vi "relay_block6.vi"(8 "error in":errorcluster, 11 "Modbus master in":refnum<class "Modbus Master.lvclass">) -> (0 "error out":errorcluster, 3 "Modbus master out":refnum<class "Modbus Master.lvclass">)   [LabVIEW 2020]
uses:
  <vilib>/NI/Modbus Library/API/Master/Modbus Master.lvclass
  C:/Program Files/National Instruments/LabVIEW 2020/vi.lib/NI/Modbus Library/API/Modbus API.lvclass
  <vilib>/NI/Modbus Library/API/Modbus API.lvclass/Modbus API.ctl
  <vilib>/NI/Modbus Library/Transmission Data Unit/Transmission Data Unit.lvclass/Transmission Data Unit.ctl
  <vilib>/NI/Modbus Library/Transmission Data Unit/Write Unit ID.vi
  <vilib>/NI/Modbus Library/API/Read Transmission Data Unit.vi
  <vilib>/NI/Modbus Library/API/Write Transmission Data Unit.vi
  status/emergency stop.vi
panel:
  out "current time":timestamp
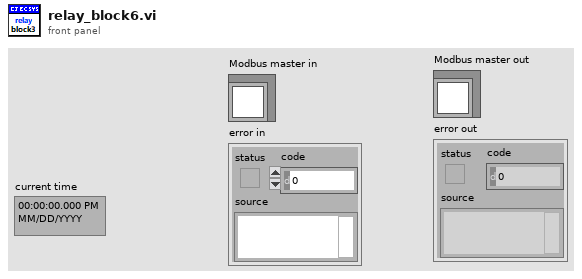
[diagram p1: front panel]
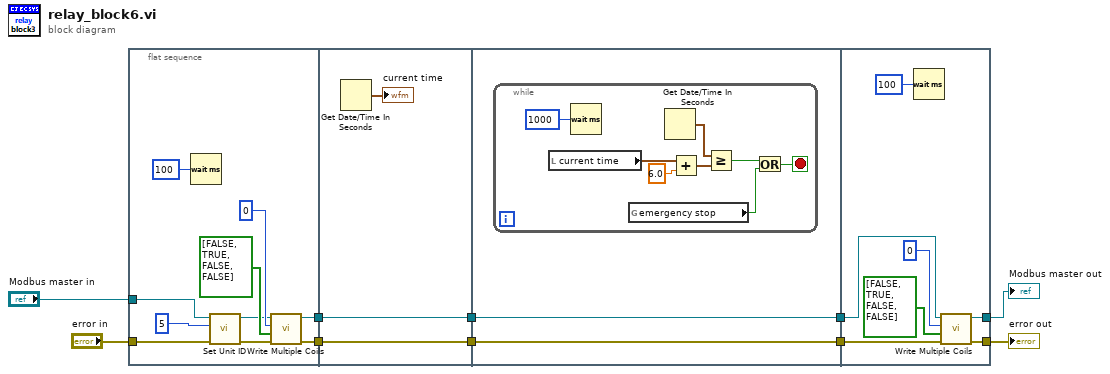
[diagram p0: block diagram]
diagram:
  n1 = flat-sequence {
    tunnel: "Modbus master in" -> [w14]
    tunnel: "error in" -> [w15]
    tunnel: [w17] -> w8
    tunnel: [w16] -> w3
    tunnel: w8 -> [w22]
    tunnel: [w22] -> w7
    tunnel: [w21] -> w4
    tunnel: w3 -> [w21]
    tunnel: w7 -> [w25]
    tunnel: [w25] -> w6
    tunnel: [w24] -> w5
    tunnel: w4 -> [w24]
    tunnel: w6 -> [w37]
    tunnel: w5 -> [w36]
    tunnel: [w35] -> w2
    tunnel: [w34] -> w1
    frame #0 {
      n2 = Wait (ms)(milliseconds to wait=u32 100 ("millisecond timer value")) -> ()  [unwired: 1 out]
      n3 = call <vilib>:"Set Unit ID.vi"("error in"=w15, "unit ID"=u8 5, "Modbus master in"=w14) -> ("error out"=w12:errorcluster, "Modbus master out"=w13:refnum<class "Modbus Master.lvclass">)  [unwired: 7 in]
      n4 = call-dynamic "Write Multiple Coils.vi"("error in"=w12, "coils to write"=bool[] [FALSE, TRUE, FALSE, FALSE] ("coils 2"), "starting address"=u16 0, "Modbus master in"=w13) -> ("error out"=w16:errorcluster, "Modbus master out"=w17:refnum<class "Modbus Master.lvclass">)  [unwired: 6 in]
    }
    frame #1 {
      n5 = Get Date/Time In Seconds() -> (seconds since 1Jan1904=→"current time":timestamp)
    }
    frame #2 {
      n6 = while {
        stop <- w26 stop-if-true
        n7 = local read "current time"() -> (w32:timestamp)
        n8 = Wait (ms)(milliseconds to wait=u32 1000 ("millisecond timer value")) -> ()  [unwired: 1 out]
        n9 = global read "emergency stop.vi" "emergency stop"() -> (w27:bool)
        n10 = Get Date/Time In Seconds() -> (seconds since 1Jan1904=w29:timestamp)
        n11 = Add(x=w32, y=6.0) -> (x+y=w30:timestamp)
        n12 = Greater Or Equal?(x=w29, y=w30) -> (x >= y?=w28:bool)
        n13 = Or(x=w28, y=w27) -> (x .or. y?=w26:bool)
      }
    }
    frame #3 {
      n14 = Wait (ms)(milliseconds to wait=u32 100 ("millisecond timer value")) -> ()  [unwired: 1 out]
      n15 = call-dynamic "Write Multiple Coils.vi"("error in"=w36, "coils to write"=bool[] [FALSE, TRUE, FALSE, FALSE] ("coils 2"), "starting address"=u16 0, "Modbus master in"=w37) -> ("error out"=w34:errorcluster, "Modbus master out"=w35:refnum<class "Modbus Master.lvclass">)  [unwired: 6 in]
    }
  }
  "Modbus master out" <- w2
  "error out" <- w1
